vi "RegisterSplit.vi"(8 "register values":u16[](array[numeric])) -> (0 "[0] Motor1On":bool, 1 "[1]Motor2On":bool, 2 "[2]StartMotor1":bool, 3 "[3]StartMotor2":bool, 4 "[4] SetSpeed1":dbl format="%.2f", 5 "[5] SetSpeed2":dbl format="%.2f", 14 "[7]ReadSpeed1":dbl format="%.2f", 15 "[8] ReadSpeed2":dbl format="%.2f", 16 "[6] MotorsOff":bool, 17 "[9]Motor1Ok":bool, 18 "[10]Motor2Ok":bool)   [LabVIEW 2024]
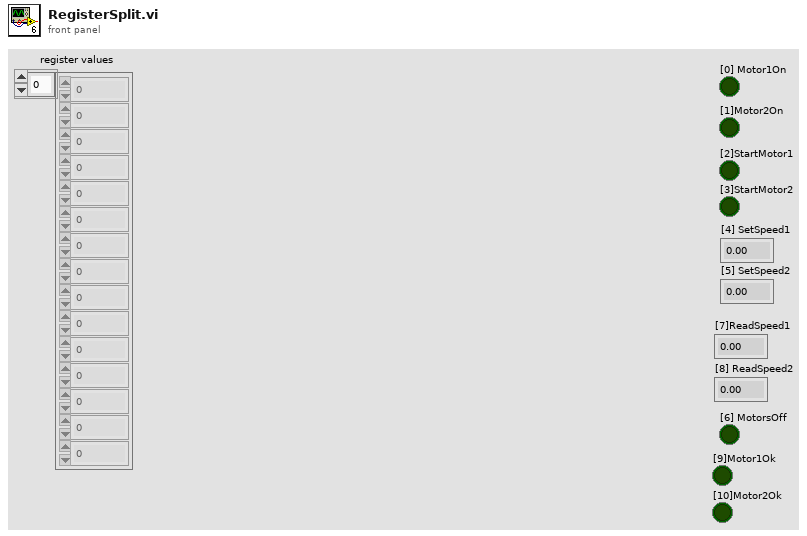
[diagram p1: front panel]
types:
  T1 = cluster{"register values[0]":u16, "register values[1]":u16, "register values[2]":u16, "register values[3]":u16, "register values[4]":u16, "register values[5]":u16, "register values[6]":u16, "register values[7]":u16, "register values[8]":u16, "register values[9]":u16, "register values[10]":u16, "register values[11]":u16, "register values[12]":u16, "register values[13]":u16, "register values[14]":u16}
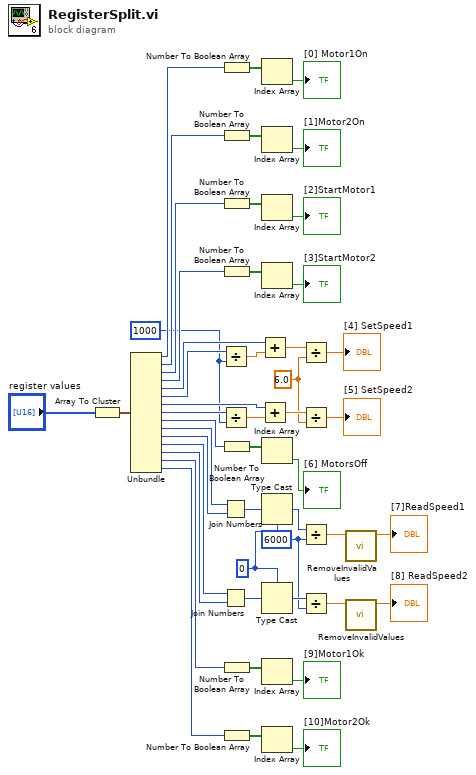
[diagram p0: block diagram]
diagram:
  w10 = 6000 ("y")
  w14 = 6.0 ("y")
  w15 = u16 1000 ("y")
  w33 = 0
  n1 = Array To Cluster(array="register values") -> (cluster=w38:T1)
  n2 = Unbundle(w38) -> ("register values[0]"=w37:u16, "register values[1]"=w36:u16, "register values[2]"=w35:u16, "register values[3]"=w34:u16, "register values[4]"=w22:u16, "register values[5]"=w24:u16, "register values[6]"=w17:u16, "register values[7]"=w16:u16, "register values[8]"=w3:u16, "register values[9]"=w5:u16, "register values[10]"=w4:u16, "register values[11]"=w2:u16, "register values[12]"=w1:u16, "register values[13]"=w28:u16, "register values[14]"=w25:u16)
  n3 = Divide(x=w24, y=w15) -> (x/y=w23:dbl)
  n4 = Divide(x=w16, y=w15) -> (x/y=w19:dbl)
  n5 = Join Numbers(hi=w5, lo=w4) -> ((hi.lo)=w32:u32)
  n6 = Join Numbers(hi=w2, lo=w1) -> ((hi.lo)=w31:u32)
  n7 = Number To Boolean Array(number=w37) -> (Boolean array=w49:bool[])
  n8 = Number To Boolean Array(number=w36) -> (Boolean array=w47:bool[])
  n9 = Number To Boolean Array(number=w35) -> (Boolean array=w45:bool[])
  n10 = Number To Boolean Array(number=w34) -> (Boolean array=w43:bool[])
  n11 = Number To Boolean Array(number=w3) -> (Boolean array=w41:bool[])
  n12 = Number To Boolean Array(number=w28) -> (Boolean array=w30:bool[])
  n13 = Number To Boolean Array(number=w25) -> (Boolean array=w27:bool[])
  n14 = Add(x=w22, y=w23) -> (x+y=w21:dbl)
  n15 = Add(x=w17, y=w19) -> (x+y=w18:dbl)
  n16 = Index Array(array=w49) -> (element=→"[0] Motor1On":bool)  [unwired: 1 in]
  n17 = Index Array(array=w47) -> (element=→"[1]Motor2On":bool)  [unwired: 1 in]
  n18 = Index Array(array=w45) -> (element=→"[2]StartMotor1":bool)  [unwired: 1 in]
  n19 = Index Array(array=w43) -> (element=→"[3]StartMotor2":bool)  [unwired: 1 in]
  n20 = Index Array(array=w41) -> (element=→"[6] MotorsOff":bool)  [unwired: 1 in]
  n21 = Type Cast(type=w33, x=w32) -> (*(type *) &x=w12:i32)
  n22 = Type Cast(type=w33, x=w31) -> (*(type *) &x=w11:i32)
  n23 = Index Array(array=w30) -> (element=→"[9]Motor1Ok":bool)  [unwired: 1 in]
  n24 = Index Array(array=w27) -> (element=→"[10]Motor2Ok":bool)  [unwired: 1 in]
  n25 = Divide(x=w21, y=w14) -> (x/y=→"[4] SetSpeed1":dbl)
  n26 = Divide(x=w18, y=w14) -> (x/y=→"[5] SetSpeed2":dbl)
  n27 = Divide(x=w12, y=w10) -> (x/y=w9:dbl)
  n28 = Divide(x=w11, y=w10) -> (x/y=w6:dbl)
  n29 = call "RemoveInvalidValues.vi"("In"=w9) -> ("Out"=→"[7]ReadSpeed1":dbl)  [unwired: 10 in]
  n30 = call "RemoveInvalidValues.vi"("In"=w6) -> ("Out"=→"[8] ReadSpeed2":dbl)  [unwired: 10 in]
